vi "Library - By Tree.vi"(7 "Msg Chain":string, 8 "error in (no error)":errorcluster {"code" format="Error %.0f"}, 10 "Libraries":refnum<class "Library Documentation.lvclass">[](array[class]), 11 "VIDoc Printer - Confluence In":refnum<class "VIDoc Printer - Confluence.lvclass">) -> (0 "error out":errorcluster {"code" format="Error %.0f"}, 3 "VIDoc Printer - Confluence Out":refnum<class "VIDoc Printer - Confluence.lvclass">)   [LabVIEW 2023, in "VIDoc Printer - Confluence.lvlib" / "VIDoc Printer - Confluence.lvclass"]
uses:
  VIDoc Printer - Confluence.lvclass
  Parsing/Library Documentation/Library Documentation.lvclass
  Confluence Formatting/Types/Format Combo Box.ctl
  VIDoc Printer - Confluence.lvclass/VIDoc Printer - Confluence.ctl
  Parsing/Library Documentation/Library Documentation.lvclass/Library Documentation.ctl
  Parsing/Library Documentation/Get Path.vi
  Accessors/Get Library By Tree Expand.vi
  Confluence Formatting/Confluence Formatting.lvlib
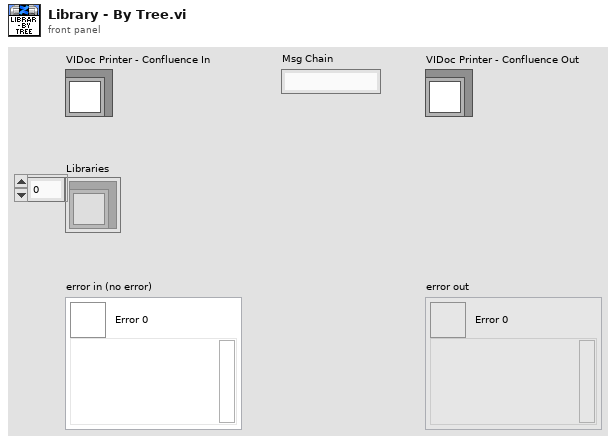
[diagram p1: front panel]
types:
  T1 = typedef "Confluence Formatting.lvlib/Format Combo Box.ctl" = string
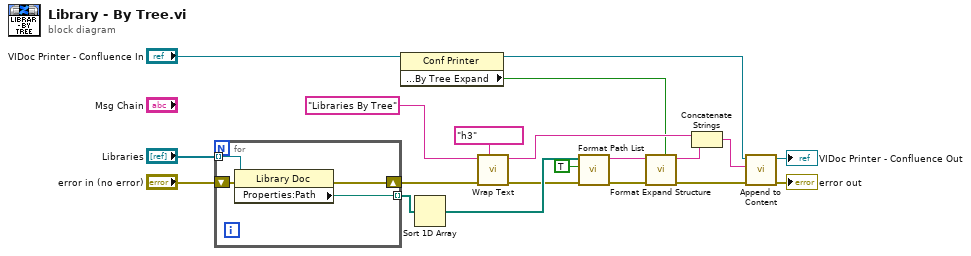
[diagram p0: block diagram]
diagram:
  n1 = for {
    tunnel: "Libraries" -> [w23] mode=indexing
    tunnel: [w21] -> w19 mode=indexing
    shift-right: [w22] -> w18
    shift-left: "error in (no error)" -> [w24]
    n2 = property class="Library Doc"(reference=w23, error in=w24) -> (error out=w22:errorcluster, "Properties:Path"=w21:path)  [unwired: 1 out]
  }
  n3 = property class="Conf Printer"(reference="VIDoc Printer - Confluence In") -> (reference out=w2:refnum<class "VIDoc Printer - Confluence.lvclass">, "Properties:Expand?:Library:By Tree Expand"=w1:bool)  [unwired: 1 in, 1 out]
  n4 = Sort 1D Array(array=w19) -> (sorted array=w15:path[])
  n5 = call "Wrap Text.vi"("Formatting"=T1 "h3", "Error in"=w18, "String"="Libraries By Tree") -> ("Error out"=w14:errorcluster, "Wrapped String"=w17:string)  [unwired: 7 in]
  n6 = call "Format Path List.vi"("Error in"=w14, "Tree (F)"=TRUE, "Paths"=w15) -> ("Error out"=w13:errorcluster, "Bullet List String"=w4:string)  [unwired: 7 in]
  n7 = call "Format Expand Structure.vi"("Enable? (T)"=w1, "Error in"=w13, "Content"=w4) -> ("Error out"=w5:errorcluster, "Expand String"=w3:string)  [unwired: 7 in]
  n8 = Concatenate Strings(w17, w3) -> (w16:string)
  n9 = call "Append to Content.vi"("error in (no error)"=w5, "Content"=w16, "VIDoc Printer - Confluence In"=w2) -> ("error out"=→"error out":errorcluster, "VIDoc Printer - Confluence Out"=→"VIDoc Printer - Confluence Out":refnum<class "VIDoc Printer - Confluence.lvclass">)  [unwired: 7 in]
